vi "Populate Photos Table.vi"() -> ()   [LabVIEW 2019]
uses:
  <vilib>/addons/database/Connection.llb/DB Tools Open Connec (String).vi
  <vilib>/addons/database/_DB Variant To Data/Database Variant To Data.xnode
  <vilib>/addons/database/NI_Database_API.lvlib
panel:
  out "Array":string[](array[string])
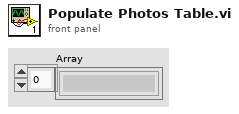
[diagram p1: front panel]
types:
  T1 = typedef "NI_Database_API.lvlib/Conn ObjectReference.ctl" = refnum<k1>
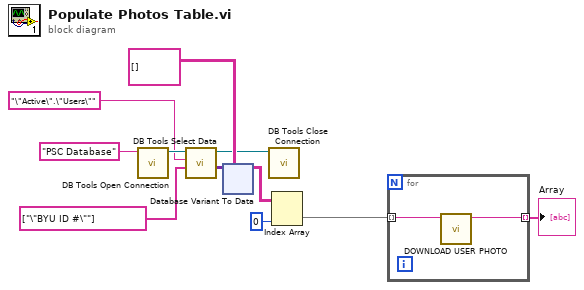
[diagram p0: block diagram]
diagram:
  n1 = call-poly <vilib>:"DB Tools Open Connection.vi"("connection information"="PSC Database") -> ("connection reference"=w10:T1)  [unwired: 7 in, 1 out]
  n2 = call <vilib>:"DB Tools Select Data.vi"("columns"=string[] ["\"BYU ID #\""], "table"="\"Active\".\"Users\"", "connection reference"=w10) -> ("data"=w7:variant[][], "connection reference out"=w6:T1)  [unwired: 3 in, 1 out]
  n3 = xnode "Database Variant To Data"("database variant"=w7, "type"=string[][] []) -> ("data"=w5:string[][])  [unwired: 1 in, 1 out]
  n4 = call <vilib>:"DB Tools Close Connection.vi"("connection reference"=w6) -> ()  [unwired: 6 in, 1 out]
  n5 = Index Array(array=w5, index (col)=0 ("disabled index (col)")) -> (element=w2:string[])  [unwired: 1 in]
  n6 = for {
    tunnel: w2 -> [w13] mode=indexing
    tunnel: [w12] -> w1 mode=indexing
    n7 = call "DOWNLOAD USER PHOTO.vi"("BYU ID #"=w13) -> ("Image String Out"=w12:string)  [unwired: 10 in]
  }
  "Array" <- w1
